vi "Write Component Operations Errors.vi"(8 "Error In":errorcluster, 10 "Component Operations Errors":errorcluster, 11 "Component in":refnum<class "Component.lvclass">) -> (0 "Error Out":errorcluster, 3 "Component out":refnum<class "Component.lvclass">)   [LabVIEW 2017, in "CL_G3_VIComponentBuilder.lvlib" / "Component.lvclass"]
uses:
  Component.lvclass
  Component.lvclass/Component.ctl
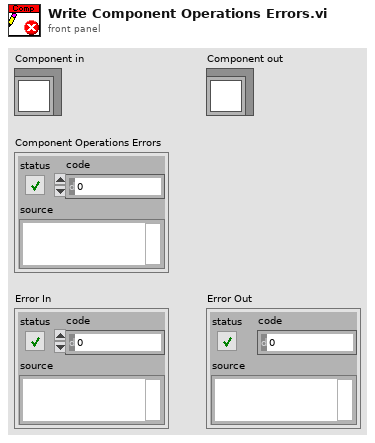
[diagram p1: front panel]
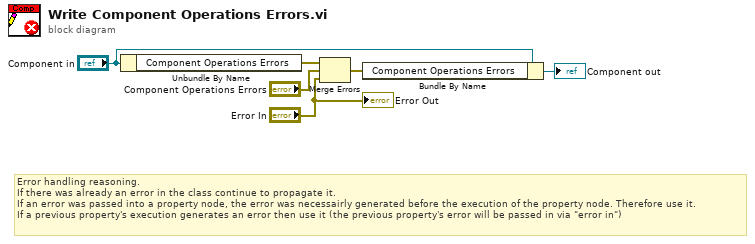
[diagram p0: block diagram]
diagram:
  # "Error handling reasoning.\nIf there was already an error in the class continue to propagate it.\nIf an error was passed into a property node, the error was necessairly generated before the execution of the property node. Therefore use it.\nIf a previous property's execution generates an error then use it (the previous property's error will be passed in via \"error in\")"
  n1 = Unbundle By Name("Component in") -> ("Component Operations Errors"=w4:errorcluster)
  n2 = Merge Errors(w4, "Component Operations Errors", "Error In") -> (w3:errorcluster)
  n3 = Bundle By Name(cluster="Component in", "Component Operations Errors"=w3) -> (→"Component out":refnum<class "Component.lvclass">)
  "Error Out" <- "Error In"
